vi "DflipFlop.vi"(8 "D":bool, 9 "Clock":bool, 10 "Reset":bool, 11 "Set":bool) -> (2 "/Q\\":bool, 3 "Q":bool)   [LabVIEW 2012]
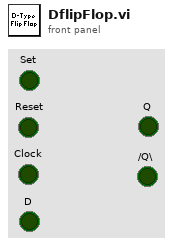
[diagram p1: front panel]
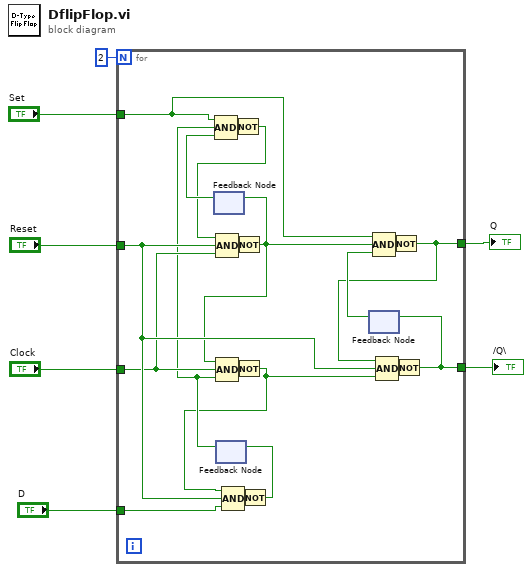
[diagram p0: block diagram]
diagram:
  n1 = for {
    N: 2 -> [_]
    tunnel: "D" -> [w20]
    tunnel: "Reset" -> [w18]
    tunnel: "Clock" -> [w17]
    tunnel: [w14] -> w4
    tunnel: "Set" -> [w13]
    tunnel: [w8] -> w2
    n2 = feedback #1() -> (w16:bool)  [unwired: 1 in]
    n3 = feedback #2() -> (w15:bool)  [unwired: 1 in]
    n4 = Compound Arithmetic op=AND(w13, w15, w16) -> (w26:bool)
    n5 = Not(x=w26) -> (.not. x?=w10:bool)
    n6 = Compound Arithmetic op=AND(w10, w18, w17) -> (w25:bool)
    n7 = Not(x=w25) -> (.not. x?=w11:bool)
    n8 = feedback-in #1(w11) -> ()
    n9 = Compound Arithmetic op=AND(w11, w17, w15) -> (w24:bool)
    n10 = Not(x=w24) -> (.not. x?=w9:bool)
    n11 = Compound Arithmetic op=AND(w9, w18, w20) -> (w23:bool)
    n12 = Not(x=w23) -> (.not. x?=w19:bool)
    n13 = feedback-in #2(w19) -> ()
    n14 = feedback #3() -> (w12:bool)  [unwired: 1 in]
    n15 = Compound Arithmetic op=AND(w13, w11, w12) -> (w21:bool)
    n16 = Not(x=w21) -> (.not. x?=w8:bool)
    n17 = Compound Arithmetic op=AND(w8, w18, w9) -> (w22:bool)
    n18 = Not(x=w22) -> (.not. x?=w14:bool)
    n19 = feedback-in #3(w14) -> ()
  }
  "Q" <- w2
  "/Q\\" <- w4
